vi "ButtonSend.vi"(8 "error in (no error)":errorcluster, 10 "Button Value":i8, 11 "Notifier Name":string="Joystick") -> (0 "error out":errorcluster)   [LabVIEW 2013]
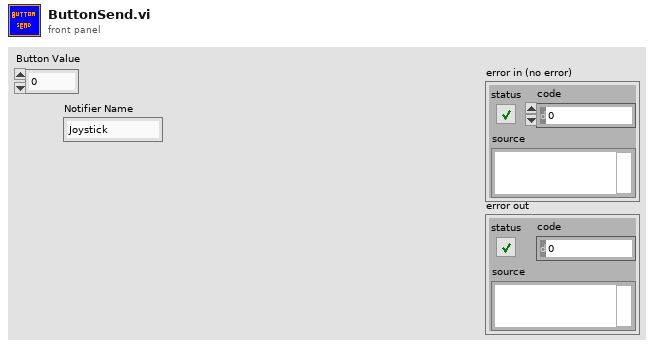
[diagram p1: front panel]
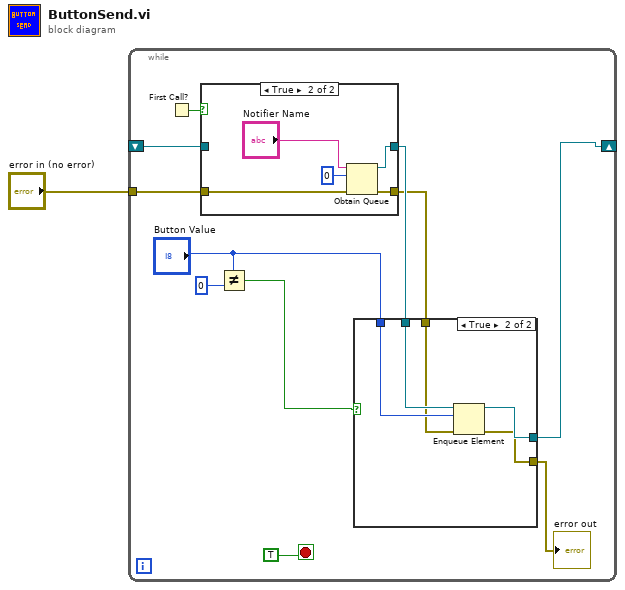
[diagram p0: block diagram]
diagram:
  n1 = while {
    shift-right: [w3] -> _
    shift-left: _ -> [w9]
    tunnel: "error in (no error)" -> [w10]
    stop <- TRUE stop-if-true
    n2 = First Call?() -> (First Call?: T/F=w11:bool)
    n3 = case shown="True" w11 {
      tunnel: [w21 w23] -> w8
      tunnel: w10 -> [w20 w24]
      tunnel: w9 -> [w21 _]
      tunnel: [w20 w22] -> w5
      frame False {
      }
      frame True {
        n4 = Obtain Queue(name (unnamed)="Notifier Name", element data type=i8 0, error in (no error)=w24) -> (queue out=w23:refnum<queue>, error out=w22:errorcluster)  [unwired: 2 in, 1 out]
      }
    }
    n5 = Not Equal?(x="Button Value", y=i8 0) -> (x != y?=w4:bool)
    n6 = case shown="True" w4 {
      tunnel: w8 -> [w13 w19]
      tunnel: "Button Value" -> [_ w18]
      tunnel: [w14 w15] -> w6
      tunnel: w5 -> [w14 w16]
      tunnel: [w13 w17] -> w3
      frame False {
      }
      frame True {
        n7 = Enqueue Element(queue=w19, element=w18, error in (no error)=w16) -> (queue out=w17:refnum<queue>, error out=w15:errorcluster)  [unwired: 1 in, 1 out]
      }
    }
    "error out" <- w6
  }
